vi "taster.vi"(1 "i":dbl, 2 "y":dbl) -> (0 "Polar Plot":picture)   [LabVIEW 2017]
panel:
  in  "Plot Color":u32(colorbox)=16715776
  in  "Grid Color":u32(colorbox)
  in  "Visible Section":u16(ring)=8
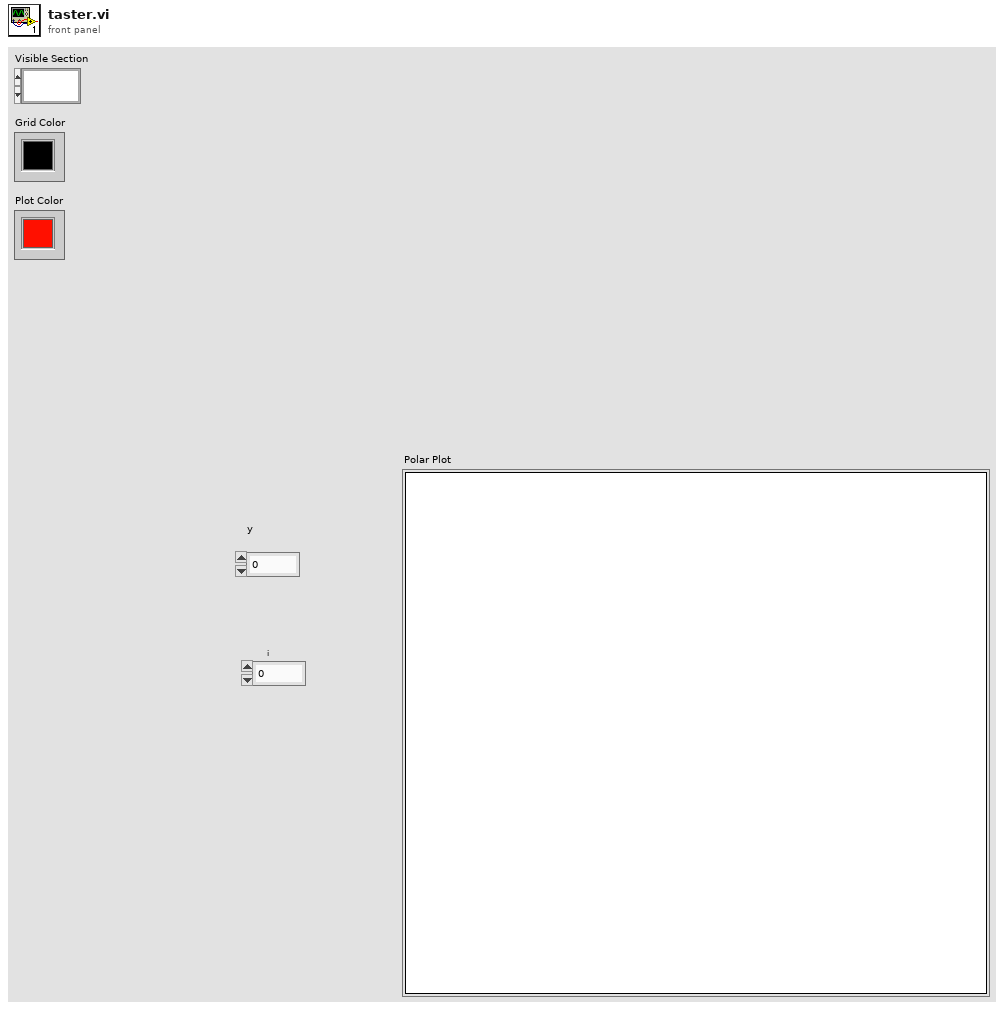
[diagram p1: front panel]
types:
  T1 = cluster{"maximum":dbl, "minimum":dbl, "clip to min":bool, "log?(F)":bool, "grid color":u32, "plot color":u32, "format and precision":cluster{"format":enum8{"Decimal", "Scientific", "Engineering", "Binary", "Octal", "Hex"}, "precision":u8}, "visible section":u16}
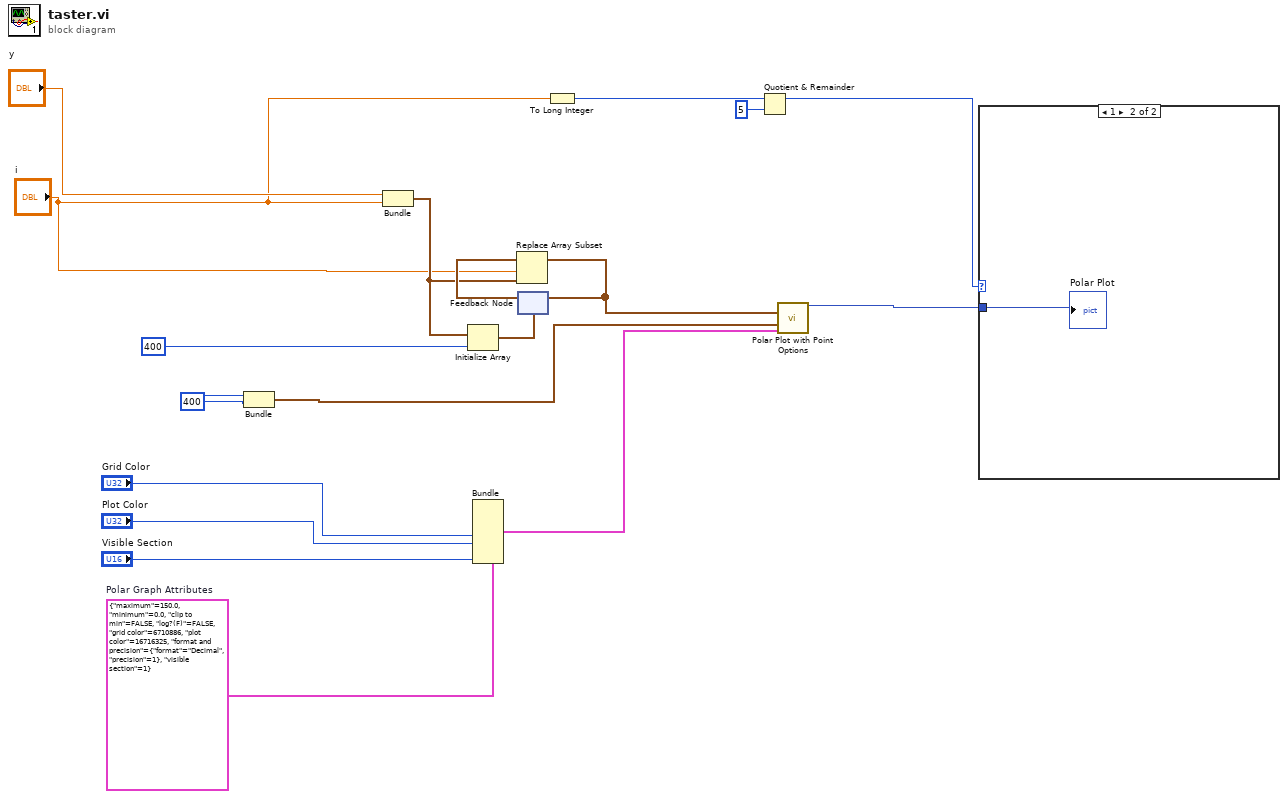
[diagram p0: block diagram]
diagram:
  w5 = u32 400
  w14 = T1 {"maximum"=150.0, "minimum"=0.0, "clip to min"=FALSE, "log?(F)"=FALSE, "grid color"=6710886, "plot color"=16716325, "format and precision"={"format"=enum."Decimal", "precision"=1}, "visible section"=1}  # Polar Graph Attributes
  n1 = Bundle(w5, w5) -> (w6:cluster{u32, u32})  [unwired: 1 in]
  n2 = Bundle("y"="y", "i"="i") -> (w15:cluster{"y\n":dbl, "i":dbl})  [unwired: 1 in]
  n3 = Initialize Array(w15, 400 ("dimension size")) -> (w17:cluster{"y\n":dbl, "i":dbl}[])
  n4 = Bundle(cluster=w14, "grid color"="Grid Color", "plot color"="Plot Color", "visible section"="Visible Section") -> (w9:T1)  [unwired: 5 in]
  n5 = feedback #1(w17) -> (w18:cluster{"y\n":dbl, "i":dbl}[])
  n6 = Replace Array Subset(array=w18, new element=w15, index="i") -> (w8:cluster{"y\n":dbl, "i":dbl}[])
  n7 = feedback-in #1(w8) -> ()
  n8 = To Long Integer(number="i") -> (32bit integer=w4:i32)
  n9 = Quotient & Remainder(x=w4, y=5) -> (x-y*floor(x/y)=w2:i32)  [unwired: 1 out]
  n10 = call <vilib>:"Polar Plot with Point Options.vi"("data array [mag, phase (deg)]"=w8, "dimensions (w,h)"=w6, "polar attributes"=w9) -> ("new picture"=w7:picture)  [unwired: 12 in]
  n11 = case shown="1" w2 {
    tunnel: w7 -> [_ w19]
    frame 0, Default {
    }
    frame 1 {
      "Polar Plot" <- w19
    }
  }
